vi "4155C Output Config SMUs v3.0.vi"(0 "VISA resource name in":refnum<visa-resource-name>, 1 "Pulse period":dbl=0.005 min=0.005 max=1.0 step=0.0001 format="%.4f", 2 "Source/Common":u32(ring) items=["SMU1  ", "SMU2  ", "SMU3  ", "SMU4  ", "SMU5  ", "SMU6  ", "VSU1  ", "VSU2  "], 3 "Pulse width":dbl=0.0005 min=0.0005 max=0.1 step=0.0001 format="%.4f", 4 "Base voltage":dbl format="%^.4e", 5 "error in (no error)":errorcluster, 6 "sweep method":u16(ring) items=["Continuous", "Pulsed"], 7 "SMU4":cluster{"on/off":bool, "Voltage":dbl} {"Voltage" min=-100.0 max=100.0 format="%.2f"}, 8 "Drain":u32(ring)=1 items=["SMU1  ", "SMU2  ", "SMU3  ", "SMU4  ", "SMU5  ", "SMU6  ", "VSU1  ", "VSU2  "], 9 "Gate":u32(ring)=2 items=["SMU1  ", "SMU2  ", "SMU3  ", "SMU4  ", "SMU5  ", "SMU6  ", "VSU1  ", "VSU2  "], 10 "Gate mode":u16(ring)=2 items=["Auto", "Limited", "Fixed"], 11 "Source/drain mode":u16(ring)=2 items=["Auto", "Limited", "Fixed"], 12 "Gate Range":u8(slide)=2 max=11 scale=0.0..11.0, 13 "Source/drain Range":u8(slide)=2 max=11 scale=0.0..11.0, 15 "Probe 4":u32(ring)=3 items=["SMU1  ", "SMU2  ", "SMU3  ", "SMU4  ", "SMU5  ", "SMU6  ", "VSU1  ", "VSU2  "], 17 "Drain Standby":bool, 18 "Gate Standby":bool) -> (14 "VISA Resource Name out":refnum<visa-resource-name>, 19 "error out":errorcluster)   [LabVIEW 2019]
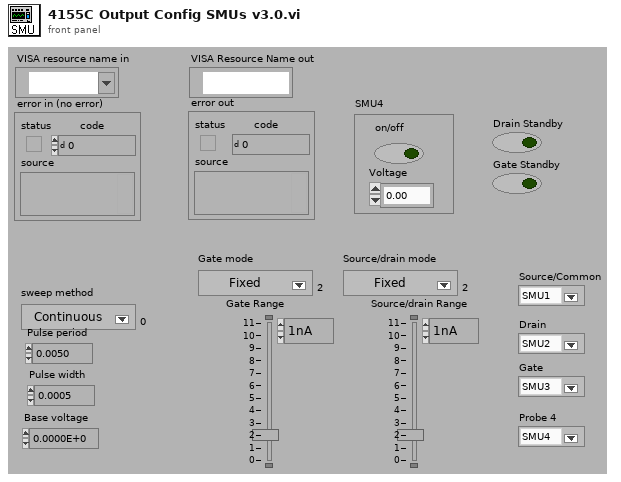
[diagram p1: front panel]
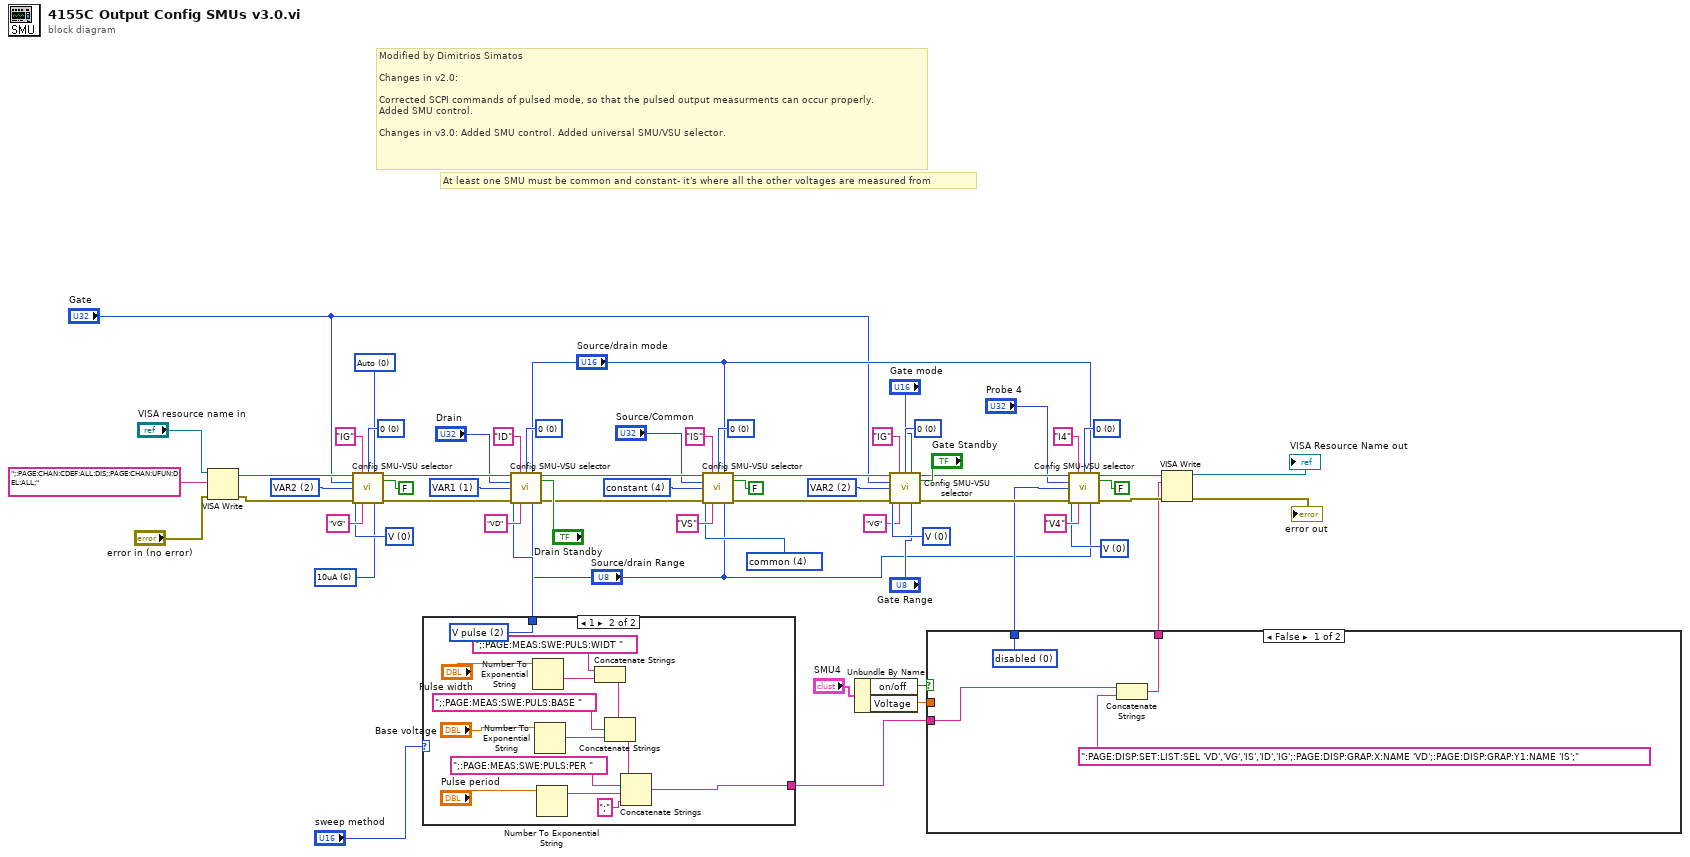
[diagram p0: block diagram]
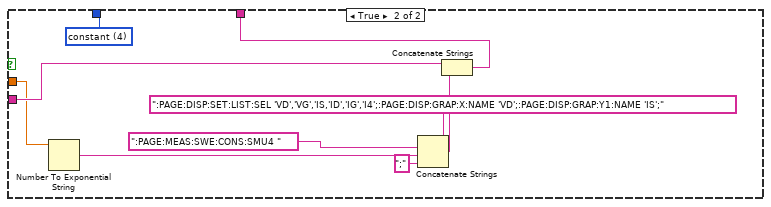
[diagram p2: hidden frame]
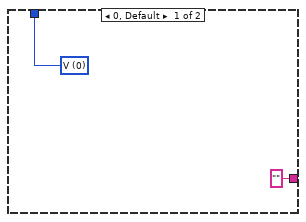
[diagram p3: hidden frame]
diagram:
  w12 = u32 0 items=["V  ", "I  ", "V pulse  ", "I pulse  ", "  common  "] ("mode")
  w19 = u16 0 items=["Auto", "Limited", "Fixed"] ("Range mode")
  w20 = u8 6 items=["10fA  ", "100fA  ", "1nA  ", "10nA", "100nA", "1uA", "10uA", "100uA", "1mA", "10mA", "100mA", "1A"] ("Range")
  w23 = u32 2 items=["disabled  ", "VAR1  ", "VAR2  ", "VAR1'  ", "constant  "] ("function")
  w25 = u32 0 items=["0  ", "10K Ohms  ", "100K Ohms  ", "1M Ohms  "] ("series resistance *")
  w26 = u32 0 items=["V  ", "I  ", "V pulse  ", "I pulse  ", "  common  "] ("mode")
  w46 = u32 0 items=["0  ", "10K Ohms  ", "100K Ohms  ", "1M Ohms  "] ("series resistance *")
  w50 = u32 0 items=["V  ", "I  ", "V pulse  ", "I pulse  ", "  common  "] ("mode")
  w51 = u32 0 items=["0  ", "10K Ohms  ", "100K Ohms  ", "1M Ohms  "] ("series resistance *")
  w53 = u32 2 items=["disabled  ", "VAR1  ", "VAR2  ", "VAR1'  ", "constant  "] ("function")
  w56 = u32 0 items=["0  ", "10K Ohms  ", "100K Ohms  ", "1M Ohms  "] ("series resistance *")
  w58 = u32 4 items=["disabled  ", "VAR1  ", "VAR2  ", "VAR1'  ", "constant  "] ("function")
  w30 = u32 4 items=["V  ", "I  ", "V pulse  ", "I pulse  ", "  common  "] ("mode")
  w61 = u32 0 items=["0  ", "10K Ohms  ", "100K Ohms  ", "1M Ohms  "] ("series resistance *")
  w63 = u32 1 items=["disabled  ", "VAR1  ", "VAR2  ", "VAR1'  ", "constant  "] ("function")
  # "Modified by Dimitrios Simatos\n\nChanges in v2.0:\n\nCorrected SCPI commands of pulsed mode, so that the pulsed output measurments can occur properly.\nAdded SMU control.\n\nChanges in v3.0: Added SMU control. Added universal SMU/VSU selector."
  # "At least one SMU must be common and constant- it's where all the other voltages are measured from"
  n1 = VISA Write(VISA resource name="VISA resource name in", write buffer=";:PAGE:CHAN:CDEF:ALL:DIS;:PAGE:CHAN:UFUN:DEL:ALL;", error in (no error)="error in (no error)") -> (VISA resource name out=w8:refnum<visa-resource-name>, error out=w9:errorcluster)  [unwired: 1 out]
  n2 = call "Config SMU-VSU selector.vi"("VISA session"=w8, "I name (max 6 chars)"="IG", "standby"=FALSE, "Range mode"=w19, "unit to configure"="Gate", "function"=w23, "mode"=w26, "error in (no error)"=w9, "V name (max 6 chars)"="VG", "series resistance *"=w25, "Range"=w20) -> ("dup VISA resource name"=w21:refnum<visa-resource-name>, "error out"=w22:errorcluster)  [unwired: 1 in, 2 out]
  n3 = case shown="1" "sweep method" {
    tunnel: [w65 w79] -> w29
    tunnel: ["" w70] -> w17
    frame 0, Default {
      w65 = u32 0 items=["V  ", "I  ", "V pulse  ", "I pulse  ", "  common  "] ("mode")
    }
    frame 1 {
      w79 = u32 2 items=["V  ", "I  ", "V pulse  ", "I pulse  ", "  common  "] ("mode")
      n4 = Number To Exponential String(number="Pulse width") -> (E-format string=w78:string)  [unwired: 3 in]
      n5 = Number To Exponential String(number="Base voltage") -> (E-format string=w74:string)  [unwired: 3 in]
      n6 = Number To Exponential String(number="Pulse period") -> (E-format string=w71:string)  [unwired: 3 in]
      n7 = Concatenate Strings(";:PAGE:MEAS:SWE:PULS:WIDT " ("Substring"), w78) -> (w76:string)
      n8 = Concatenate Strings(w76, ";:PAGE:MEAS:SWE:PULS:BASE " ("Substring"), w74) -> (w72:string)
      n9 = Concatenate Strings(w72, ";:PAGE:MEAS:SWE:PULS:PER " ("Substring"), w71, ";" ("Substring")) -> (w70:string)
    }
  }
  n10 = call "Config SMU-VSU selector.vi"("VISA session"=w21, "I name (max 6 chars)"="ID", "standby"="Drain Standby", "Range mode"="Source/drain mode", "unit to configure"="Drain", "function"=w63, "mode"=w29, "error in (no error)"=w22, "V name (max 6 chars)"="VD", "series resistance *"=w61, "Range"="Source/drain Range") -> ("dup VISA resource name"=w43:refnum<visa-resource-name>, "error out"=w42:errorcluster)  [unwired: 1 in, 2 out]
  n11 = call "Config SMU-VSU selector.vi"("VISA session"=w43, "I name (max 6 chars)"="IS", "standby"=FALSE, "Range mode"="Source/drain mode", "unit to configure"="Source/Common", "function"=w58, "mode"=w30, "error in (no error)"=w42, "V name (max 6 chars)"="VS", "series resistance *"=w56, "Range"="Source/drain Range") -> ("dup VISA resource name"=w40:refnum<visa-resource-name>, "error out"=w41:errorcluster)  [unwired: 1 in, 2 out]
  n12 = Unbundle By Name("SMU4") -> ("on/off"=w16:bool, "Voltage"=w14:dbl)
  n13 = call "Config SMU-VSU selector.vi"("VISA session"=w40, "I name (max 6 chars)"="IG", "standby"="Gate Standby", "Range mode"="Gate mode", "unit to configure"="Gate", "function"=w53, "mode"=w50, "error in (no error)"=w41, "V name (max 6 chars)"="VG", "series resistance *"=w51, "Range"="Gate Range") -> ("dup VISA resource name"=w39:refnum<visa-resource-name>, "error out"=w38:errorcluster)  [unwired: 1 in, 2 out]
  n14 = case shown="False" w16 {
    tunnel: w17 -> [w82 w92]
    tunnel: [w81 w91] -> w15
    tunnel: w14 -> [_ w89]
    tunnel: [w80 w90] -> w13
    frame False {
      w80 = u32 0 items=["disabled  ", "VAR1  ", "VAR2  ", "VAR1'  ", "constant  "] ("function")
      n15 = Concatenate Strings(w82, ":PAGE:DISP:SET:LIST:SEL 'VD','VG','IS','ID','IG';:PAGE:DISP:GRAP:X:NAME 'VD';:PAGE:DISP:GRAP:Y1:NAME 'IS';" ("write buffer (\"\")")) -> (w81:string)
    }
    frame True {
      w90 = u32 4 items=["disabled  ", "VAR1  ", "VAR2  ", "VAR1'  ", "constant  "] ("function")
      n16 = Number To Exponential String(number=w89) -> (E-format string=w87:string)  [unwired: 3 in]
      n17 = Concatenate Strings(":PAGE:DISP:SET:LIST:SEL 'VD','VG','IS,'ID','IG','I4';:PAGE:DISP:GRAP:X:NAME 'VD';:PAGE:DISP:GRAP:Y1:NAME 'IS';" ("write buffer (\"\")"), ":PAGE:MEAS:SWE:CONS:SMU4 " ("write buffer (\"\")"), w87, ";" ("Substring")) -> (w85:string)
      n18 = Concatenate Strings(w92, w85) -> (w91:string)
    }
  }
  n19 = call "Config SMU-VSU selector.vi"("VISA session"=w39, "I name (max 6 chars)"="I4", "standby"=FALSE, "Range mode"="Source/drain mode", "unit to configure"="Probe 4", "function"=w13, "mode"=w12, "error in (no error)"=w38, "V name (max 6 chars)"="V4", "series resistance *"=w46, "Range"="Source/drain Range") -> ("dup VISA resource name"=w37:refnum<visa-resource-name>, "error out"=w36:errorcluster)  [unwired: 1 in, 2 out]
  n20 = VISA Write(VISA resource name=w37, write buffer=w15, error in (no error)=w36) -> (VISA resource name out=→"VISA Resource Name out":refnum<visa-resource-name>, error out=→"error out":errorcluster)  [unwired: 1 out]
